vi "Init_LotObj.vi"(8 "error in (no error)":errorcluster, 11 "WaferTablle_Ref":refnum<vi>) -> (0 "error out":errorcluster, 3 "LotData out":refnum<class "LotData.lvclass">)   [LabVIEW 2012, in "LotData.lvclass"]
uses:
  LotData.lvclass
  Controls/TestData.ctl
  Controls/WaferTable.ctl
  LotData.lvclass/LotData.ctl
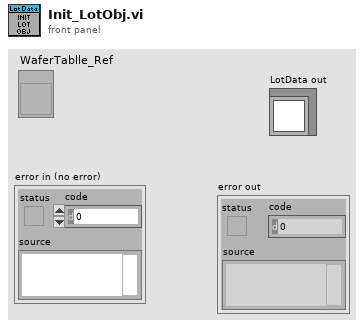
[diagram p1: front panel]
types:
  T1 = cluster{"Area":string, "Wavelength":dbl[], "EL Spectrum":dbl[]}
  T2 = typedef "TestData.ctl" = cluster{"20mA Data":cluster{"Area":string, "Current,mA":dbl, "Power":dbl, "WL":dbl, "Voltage":dbl, "Knee Current":dbl, "Reverse":dbl}, "50mA Data":cluster{"Area":string, "Current,mA":dbl, "Power":dbl, "WL":dbl, "Voltage":dbl}}
  T3 = typedef "WaferTable.ctl" = string[][]
  T4 = cluster{"Area":string, "Current,mA":dbl, "Power":dbl, "WL":dbl, "Voltage":dbl, "Knee Current":dbl, "Reverse":dbl}
  T5 = cluster{"Area":string, "Current,mA":dbl, "Power":dbl, "WL":dbl, "Voltage":dbl}
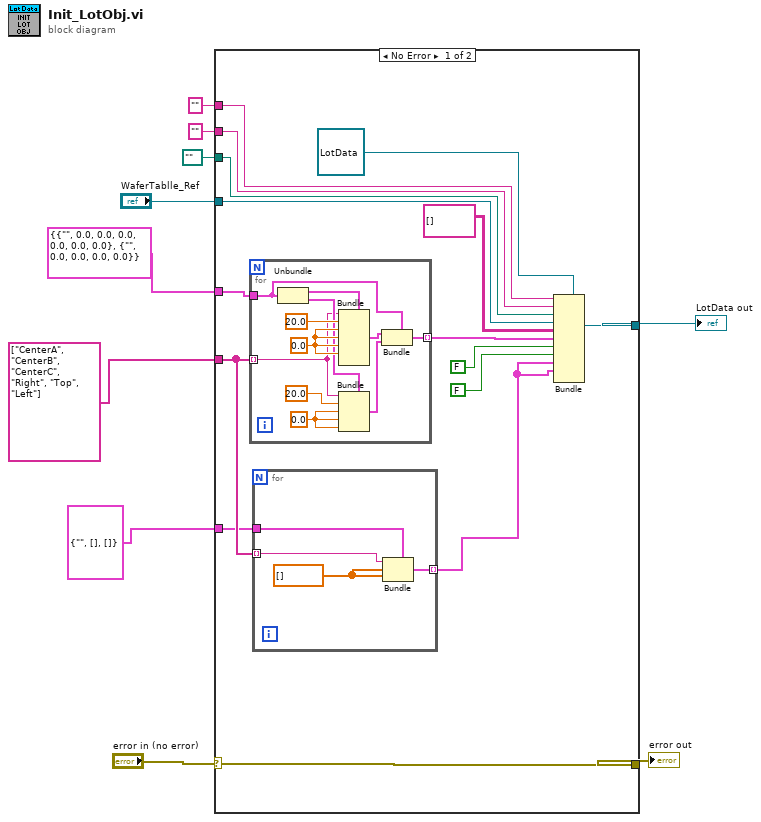
[diagram p0: block diagram]
diagram:
  n1 = case shown="No Error" "error in (no error)" {
    selector: "error in (no error)" -> [w25 w41]
    tunnel: [w25 w41] -> w9
    tunnel: [w21 _] -> w8
    tunnel: "" ("Wafer ID") -> [w24 _]
    tunnel: "" ("Type") -> [w23 _]
    tunnel: path "" ("FilePath") -> [w22 _]
    tunnel: string[] ["CenterA", "CenterB", "CenterC", "Right", "Top", "Left"] -> [w13 _]
    tunnel: "WaferTablle_Ref" -> [w19 _]
    tunnel: T2 {"20mA Data"={"Area"="", "Current,mA"=0.0, "Power"=0.0, "WL"=0.0, "Voltage"=0.0, "Knee Current"=0.0, "Reverse"=0.0}, "50mA Data"={"Area"="", "Current,mA"=0.0, "Power"=0.0, "WL"=0.0, "Voltage"=0.0}} ("TestData") -> [w14 _]
    tunnel: T1 {"Area"="", "Wavelength"=[], "EL Spectrum"=[]} ("Spect") -> [w12 _]
    frame No Error {
      n2 = for {
        tunnel: w14 -> [w33]
        tunnel: w13 -> [w34] mode=indexing
        tunnel: [w30] -> w20 mode=indexing
        w37 = 0.0 ("Power")
        w38 = 0.0 ("Power")
        n3 = Unbundle(w33) -> ("20mA Data"=w40:T4, "50mA Data"=w35:T5)
        n4 = Bundle(cluster=w40, "Area"=w34, "Current,mA"=20.0, "Power"=w38, "WL"=w38, "Voltage"=w38, "Knee Current"=w38) -> (w32:T4)  [unwired: 1 in]
        n5 = Bundle(cluster=w35, "Area"=w34, "Current,mA"=20.0, "Power"=w37, "WL"=w37, "Voltage"=w37) -> (w31:T5)
        n6 = Bundle(cluster=w33, "20mA Data"=w32, "50mA Data"=w31) -> (w30:T2)
      }
      n7 = for {
        tunnel: w13 -> [w28] mode=indexing
        tunnel: w12 -> [w29]
        tunnel: [w26] -> w11 mode=indexing
        w27 = dbl[] [] ("Wavelength")
        n8 = Bundle(cluster=w29, "Area"=w28, "Wavelength"=w27, "EL Spectrum"=w27) -> (w26:T1)
      }
      n9 = Bundle(cluster=refnum<class "LotData.lvclass"> refnum ("LotData out"), w24, w23, w22, w19, T3 [] ("WaferTable"), w20, FALSE ("Loaded"), FALSE ("Saved"), w11, w11) -> (w21:refnum<class "LotData.lvclass">)  [unwired: 1 in]
    }
    frame Error {
    }
  }
  "error out" <- w9
  "LotData out" <- w8
